vi "OpenAlarmFiles.vi"() -> ()   [LabVIEW 2018]
uses:
  <vilib>/addons/h5labview2/file/H5Fmode.ctl
  <vilib>/addons/h5labview2/file/H5F.lvlib
  <vilib>/addons/h5labview2/group/H5G.lvlib
  <vilib>/addons/h5labview2/dataset/H5Dread.llb/H5Dread.xnode
  <vilib>/addons/h5labview2/dataset/H5D.lvlib
  HDF5/AI_alarm_data_cluster.ctl
  HDF5/HDF5_TC_Errors.ctl
  <vilib>/addons/h5labview2/base/H5Equery.vi
  HDF5/lib_path_mod_20200519.vi
panel:
  out "error out":errorcluster
  out "AI_Alarms":T1[](array[typedef])
  out "TC_Alarms":T2[](array[typedef])
  out "names":string[](array[string])
  in  "path":path
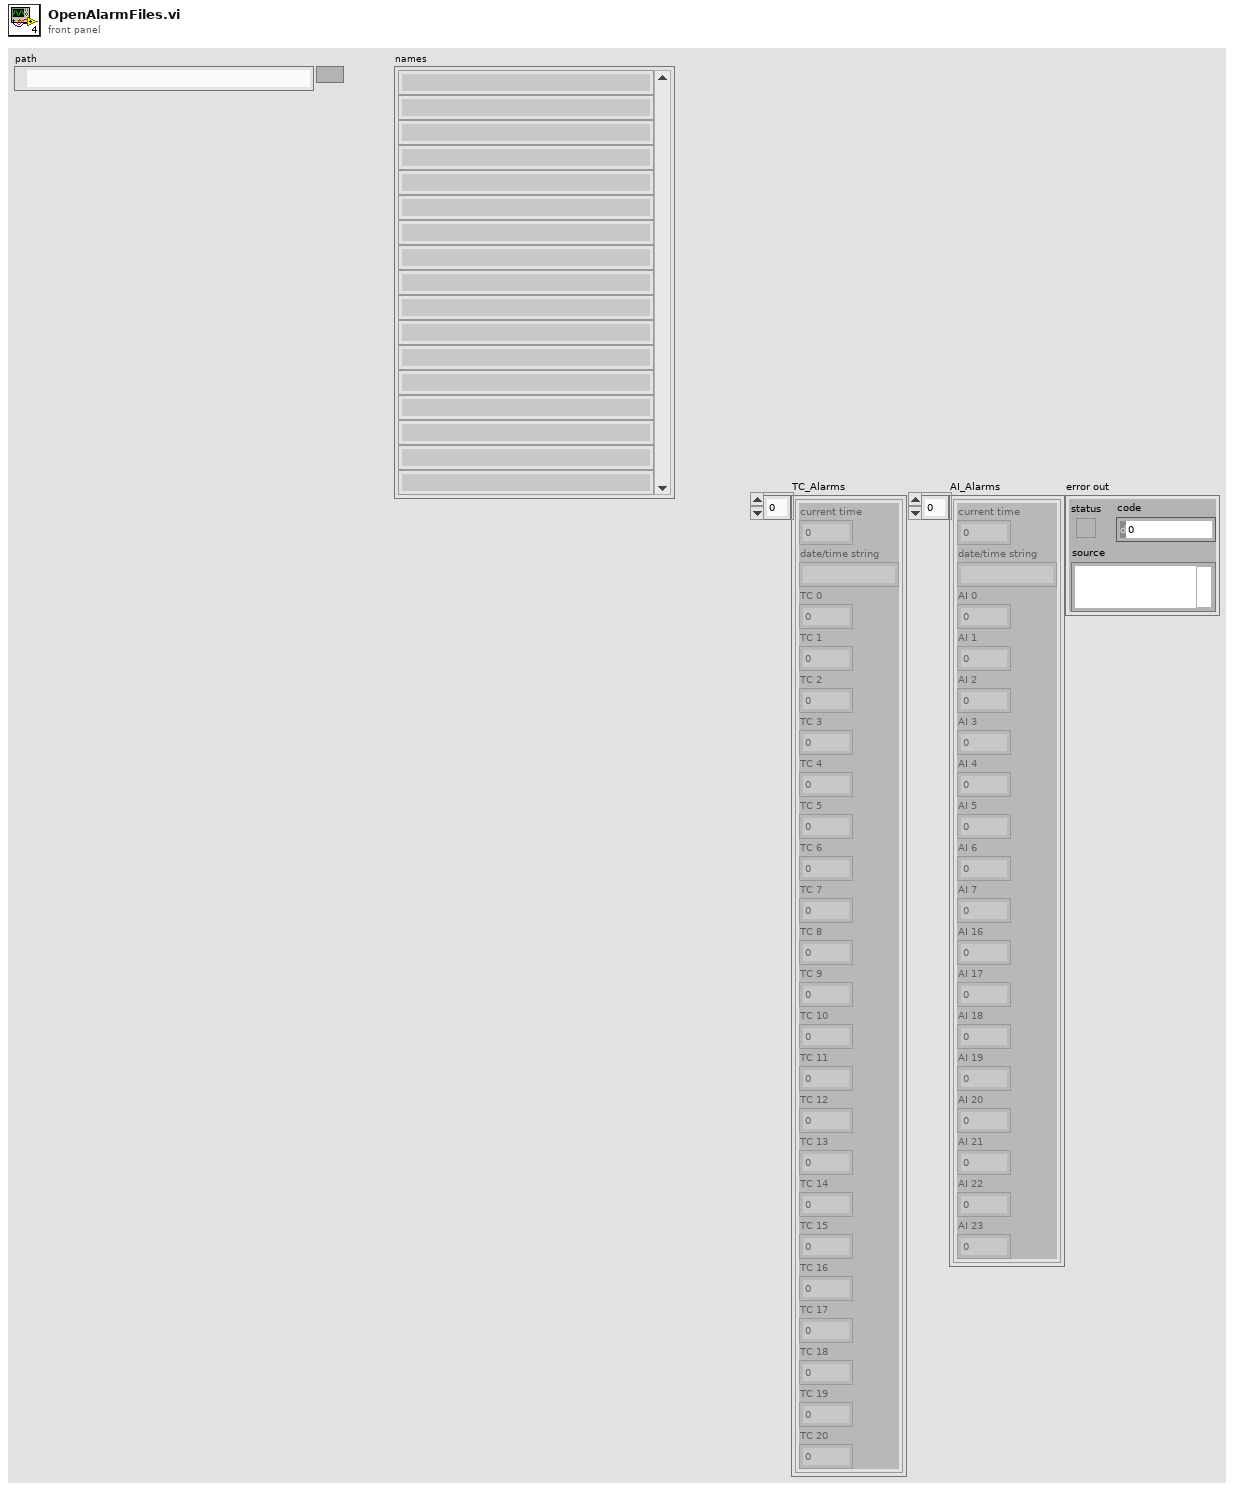
[diagram p1: front panel]
types:
  T1 = typedef "AI_alarm_data_cluster.ctl" = cluster{"current time":dbl, "date/time string":string, "AI 0":dbl, "AI 1":dbl, "AI 2":dbl, "AI 3":dbl, "AI 4":dbl, "AI 5":dbl, "AI 6":dbl, "AI 7":dbl, "AI 16":dbl, "AI 17":dbl, "AI 18":dbl, "AI 19":dbl, "AI 20":dbl, "AI 21":dbl, "AI 22":dbl, "AI 23":dbl}
  T2 = typedef "HDF5_TC_Errors.ctl" = cluster{"current time":dbl, "date/time string":string, "TC 0":dbl, "TC 1":dbl, "TC 2":dbl, "TC 3":dbl, "TC 4":dbl, "TC 5":dbl, "TC 6":dbl, "TC 7":dbl, "TC 8":dbl, "TC 9":dbl, "TC 10":dbl, "TC 11":dbl, "TC 12":dbl, "TC 13":dbl, "TC 14":dbl, "TC 15":dbl, "TC 16":dbl, "TC 17":dbl, "TC 18":dbl, "TC 19":dbl, "TC 20":dbl}
  T3 = typedef "H5F.lvlib/H5Fmode.ctl" = enum16{"read-only", "read-write", "overwrite", "create new", "open or create"}
  T4 = typedef "hid_t.ctl" = i32
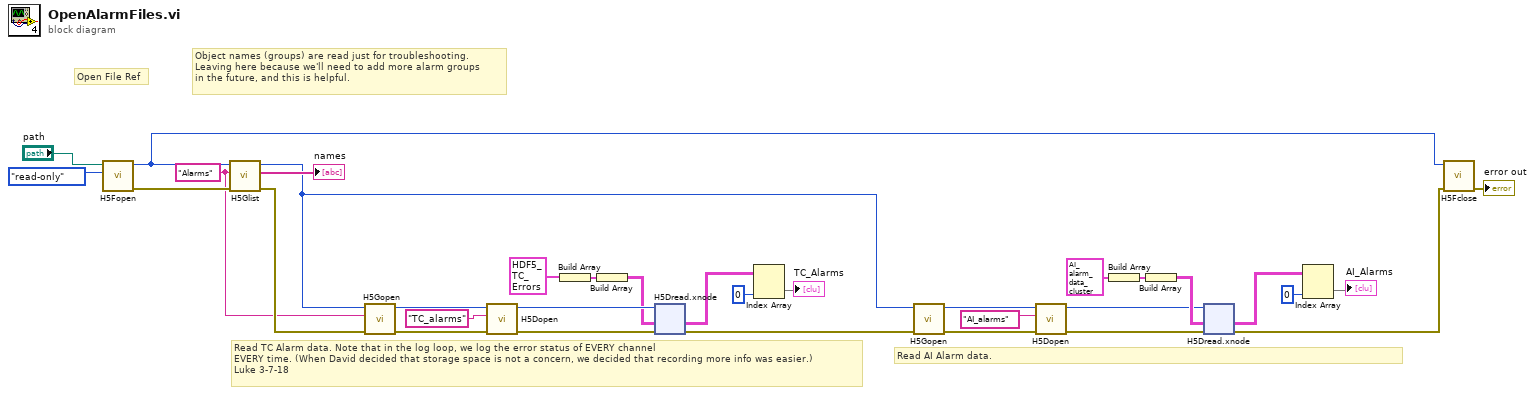
[diagram p0: block diagram]
diagram:
  w29 = "Alarms" ("group (.)")
  # "Read AI Alarm data."
  # "Read TC Alarm data. Note that in the log loop, we log the error status of EVERY channel \nEVERY time. (When David decided that storage space is not a concern, we decided that recording more info was easier.)\nLuke 3-7-18"
  # "Object names (groups) are read just for troubleshooting.\nLeaving here because we'll need to add more alarm groups\nin the future, and this is helpful."
  # "Open File Ref"
  n1 = call <vilib>:"H5Fopen.vi"("mode (read-only)"=H5Fmode."read-only" ("mode"), "path"="path") -> ("error out"=w33:errorcluster, "ref out"=w4:T4)  [unwired: 8 in]
  n2 = call <vilib>:"H5Glist.vi"("error in (no error)"=w33, "group (.)"=w29, "ref in"=w4) -> ("error out"=w30:errorcluster, "names"=→"names":string[], "ref out"=w3:T4)  [unwired: 5 in, 1 out]
  n3 = call <vilib>:"H5Gopen.vi"("error in (no error)"=w30, "name"=w29, "ref in"=w3) -> ("error out"=w26:errorcluster, "group out"=w28:T4)  [unwired: 7 in]
  n4 = call <vilib>:"H5Dopen.vi"("error in (no error)"=w26, "name"="TC_alarms" ("string"), "loc in"=w28) -> ("error out"=w25:errorcluster, "dset out"=w27:T4)  [unwired: 7 in]
  n5 = Build Array(T2 {"current time"=0.0, "date/time string"="", "TC 0"=0.0, "TC 1"=0.0, "TC 2"=0.0, "TC 3"=0.0, "TC 4"=0.0, "TC 5"=0.0, "TC 6"=0.0, "TC 7"=0.0, "TC 8"=0.0, "TC 9"=0.0, "TC 10"=0.0, "TC 11"=0.0, "TC 12"=0.0, "TC 13"=0.0, "TC 14"=0.0, "TC 15"=0.0, "TC 16"=0.0, "TC 17"=0.0, "TC 18"=0.0, "TC 19"=0.0, "TC 20"=0.0} ("TC_Alarms")) -> (w22:T2[])
  n6 = Build Array(w22) -> (w20:T2[][])
  n7 = xnode "H5Dread.xnode"("error in (no error)"=w25, "default"=w20, "ref in"=w27) -> ("error out"=w8:errorcluster, "data"=w18:T2[][])  [unwired: 3 in, 2 out]
  n8 = Index Array(array=w18, index (col)=0 ("disabled index (col)")) -> (element=→"TC_Alarms":T2[])  [unwired: 1 in]
  n9 = call <vilib>:"H5Gopen.vi"("error in (no error)"=w8, "ref in"=w3) -> ("error out"=w11:errorcluster, "group out"=w9:T4)  [unwired: 8 in]
  n10 = call <vilib>:"H5Dopen.vi"("error in (no error)"=w11, "name"="AI_alarms" ("string"), "loc in"=w9) -> ("error out"=w12:errorcluster, "dset out"=w10:T4)  [unwired: 7 in]
  n11 = Build Array(T1 {"current time"=0.0, "date/time string"="", "AI 0"=0.0, "AI 1"=0.0, "AI 2"=0.0, "AI 3"=0.0, "AI 4"=0.0, "AI 5"=0.0, "AI 6"=0.0, "AI 7"=0.0, "AI 16"=0.0, "AI 17"=0.0, "AI 18"=0.0, "AI 19"=0.0, "AI 20"=0.0, "AI 21"=0.0, "AI 22"=0.0, "AI 23"=0.0} ("AI_alarm_Clust")) -> (w13:T1[])
  n12 = Build Array(w13) -> (w14:T1[][])
  n13 = xnode "H5Dread.xnode"("error in (no error)"=w12, "default"=w14, "ref in"=w10) -> ("error out"=w7:errorcluster, "data"=w16:T1[][])  [unwired: 3 in, 2 out]
  n14 = Index Array(array=w16, index (col)=0 ("disabled index (col)")) -> (element=→"AI_Alarms":T1[])  [unwired: 1 in]
  n15 = call <vilib>:"H5Fclose.vi"("error in (no error)"=w7, "ref"=w4) -> ("error out"=→"error out":errorcluster)  [unwired: 9 in]
